vi "Get Humidity.vi"(8 "error in":errorcluster, 10 "Dew Point Scale":T1, 11 "Michell Easydew in":refnum<class "Michell Easidew.lvclass">) -> (0 "error out":errorcluster, 1 "Relative Humidity":dbl, 2 "Dew Point":dbl=-1.0, 3 "Michell Easydew out":refnum<class "Michell Easidew.lvclass">, 4 "Gas Temperature":dbl, 6 "Temperature Scale":T1)   [LabVIEW 2011, in "Michell Easidew.lvclass"]
uses:
  Michell Easidew.lvclass
  Dew Point Scale.ctl
  Michell Easidew.lvclass/Michell Easidew.ctl
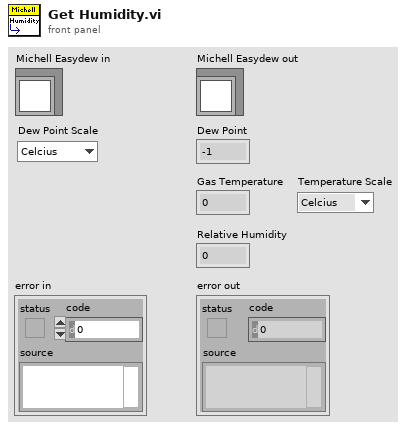
[diagram p1: front panel]
types:
  T1 = typedef "Michell Easidew.lvclass/Dew Point Scale.ctl" = enum16{"Celcius", "Fahrenheit"}
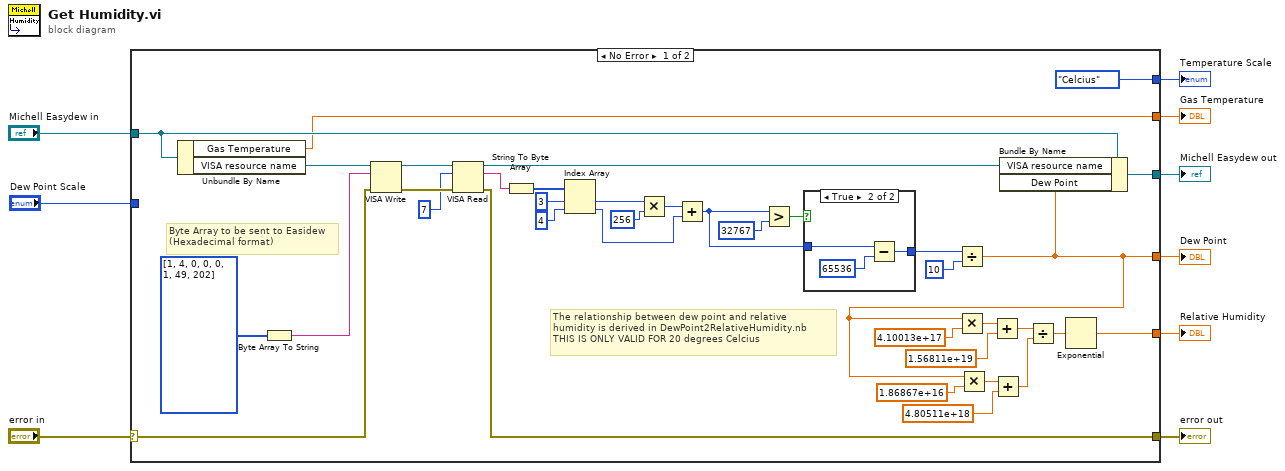
[diagram p0: block diagram]
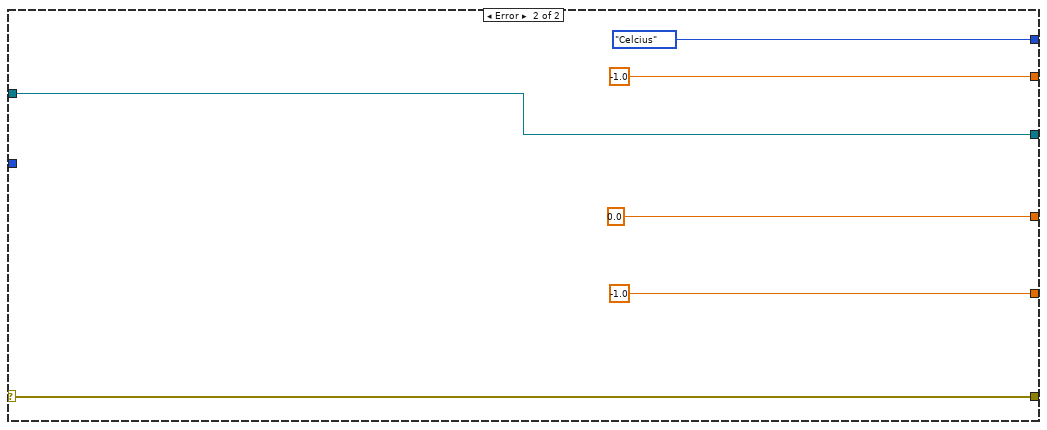
[diagram p3: hidden frame]
diagram:
  n1 = case shown="No Error" "error in" {
    selector: "error in" -> [w43 w56]
    tunnel: [w39 w56] -> w8
    tunnel: [w36 w55] -> w6
    tunnel: "Michell Easydew in" -> [w38 w55]
    tunnel: "Dew Point Scale" -> [_ _]
    tunnel: [w12 0.0] -> w4
    tunnel: [Dew_Point_Scale."Celcius" ("Dew Point Scale") Dew_Point_Scale."Celcius" ("Dew Point Scale")] -> w3
    tunnel: [w11 -1.0] -> w2
    tunnel: [w10 -1.0 ("Gas Temperature")] -> w1
    frame No Error {
      # "The relationship between dew point and relative\nhumidity is derived in DewPoint2RelativeHumidity.nb\nTHIS IS ONLY VALID FOR 20 degrees Celcius"
      # "Byte Array to be sent to Easidew\n(Hexadecimal format)"
      n2 = Unbundle By Name(w38) -> ("Gas Temperature"=w10:dbl, "VISA resource name"=w45:refnum<visa-resource-name>)
      n3 = Byte Array To String(unsigned byte array=u8[] [1, 4, 0, 0, 0, 1, 49, 202]) -> (string=w44:string)
      n4 = VISA Write(VISA resource name=w45, write buffer=w44, error in (no error)=w43) -> (VISA resource name out=w42:refnum<visa-resource-name>, error out=w41:errorcluster)  [unwired: 1 out]
      n5 = VISA Read(VISA resource name=w42, byte count=u32 7, error in (no error)=w41) -> (VISA resource name out=w37:refnum<visa-resource-name>, read buffer=w35:string, error out=w39:errorcluster)  [unwired: 1 out]
      n6 = String To Byte Array(string=w35) -> (unsigned byte array=w34:u8[])
      n7 = Index Array(array=w34, index #1=3 ("index"), index #2=4 ("index")) -> (element #1=w29:u8, element #2=w23:u8)
      n8 = Multiply(x=w29, y=256) -> (x*y=w30:i32)
      n9 = Add(x=w30, y=w23) -> (x+y=w26:i32)
      n10 = Greater?(x=w26, y=i16 32767) -> (0:w27:bool)
      n11 = case shown="True" w27 {
        tunnel: w26 -> [w47 w50]
        tunnel: [w47 w48] -> w25
        frame False {
        }
        frame True {
          n12 = Subtract(x=w50, y=65536) -> (x-y=w48:i32)
        }
      }
      n13 = Divide(x=w25, y=i16 10) -> (x/y=w12:dbl)
      n14 = Multiply(x=w12, y=4.10013e+17) -> (x*y=w17:dbl)
      n15 = Multiply(x=w12, y=1.86867e+16) -> (x*y=w19:dbl)
      n16 = Add(x=w17, y=1.56811e+19) -> (x+y=w15:dbl)
      n17 = Add(x=w19, y=4.80511e+18) -> (x+y=w14:dbl)
      n18 = Bundle By Name(cluster=w38, "VISA resource name"=w37, "Dew Point"=w12) -> (w36:refnum<class "Michell Easidew.lvclass">)
      n19 = Divide(x=w15, y=w14) -> (x/y=w13:dbl)
      n20 = Exponential(1:w13) -> (0:w11:dbl)
    }
    frame Error {
    }
  }
  "error out" <- w8
  "Michell Easydew out" <- w6
  "Dew Point" <- w4
  "Temperature Scale" <- w3
  "Relative Humidity" <- w2
  "Gas Temperature" <- w1
